vi "getExchangeBoundQueue.vi"(8 "error in (no error)":errorcluster, 9 "routingKey":string, 10 "exchangeName":string, 11 "RabbitMQ Config":T1) -> (0 "error out":errorcluster, 3 "RabbitMQ Session Out":T2)   [LabVIEW 2019, in "rabbitmq.lvlib"]
uses:
  rabbitmq.lvlib
  session.ctl
  config.ctl
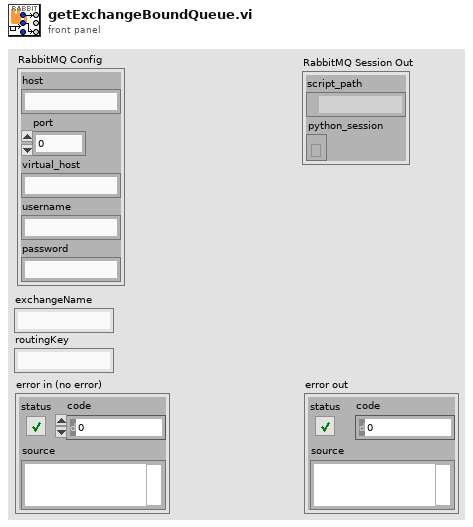
[diagram p1: front panel]
types:
  T1 = typedef "rabbitmq.lvlib/config.ctl" = cluster{"host":string, "port":i32, "virtual_host":string, "username":string, "password":string}
  T2 = typedef "rabbitmq.lvlib/session.ctl" = cluster{"script_path":path, "python_session":refnum<k35>}
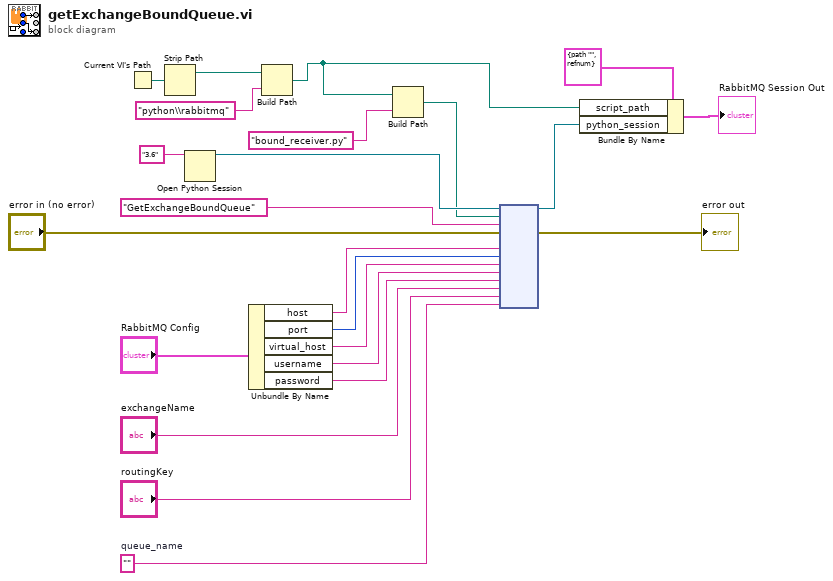
[diagram p0: block diagram]
diagram:
  w1 = ""  # queue_name
  n1 = Current VI's Path() -> (path=w8:path)
  n2 = Strip Path(path=w8) -> (stripped path=w7:path)  [unwired: 1 out]
  n3 = Open Python Session(python version="3.6" ("Python version")) -> (session out=w12:refnum<k35>)  [unwired: 2 in, 1 out]
  n4 = Unbundle By Name("RabbitMQ Config") -> ("host"=w16:string, "port"=w17:i32, "virtual_host"=w18:string, "username"=w19:string, "password"=w20:string)
  n5 = Build Path(base path=w7, name or relative path="python\\rabbitmq") -> (appended path=w6:path)
  n6 = Build Path(base path=w6, name or relative path="bound_receiver.py") -> (appended path=w4:path)
  n7 = node(w12, w4, "GetExchangeBoundQueue" ("function name"), "error in (no error)", w16, w17, w18, w19, w20, "exchangeName", "routingKey", w1) -> (w22:refnum<k35>, →"error out":errorcluster)  [unwired: 10 in, 2 out]
  n8 = Bundle By Name(cluster=T2 {"script_path"=path "", "python_session"=refnum}, "script_path"=w6, "python_session"=w22) -> (→"RabbitMQ Session Out":T2)
